vi "PH_VacuumControl.panel.vi"(0 "object ref":refnum<vi>, 5 "error in (no error)":errorcluster) -> (19 "error out":errorcluster)   [LabVIEW 2014, in "PH_VacuumControl.lvlib"]
doc: "By this VI a ross relais can be monitored and switched. \n\nThe indicators \"CLOSED\", \"OPEN\" and \"SWITCH STATE\" show the value of the Beckhoff-Tag: blue indicates bad tag status reference problems, darkgreen false and lightgreen on. If everything is working fine, \"CLOSED\" and \"SWITCH STATE\" should show the same value, while \"OPEN\" has the opposite value. \n\nThe oval button switches the ross relais. It should be in the same state as the \"SWITCH STATE\" indicator. \n\n\"EXIT\" closes the front panel (GUI), while \"Delete Instance\" disconnects and removes the instance from the PCS.\n\nThis VI has no machine safety relevant logig: there is neither a check of internal conclict nor with other objects, for example conflict with other ross relais. Therefore it must be handled with care and should be operated by well educated operators only. It is forseen exclusively for direct operating and testing of the system. \n\nLicense Agreement for this software:\n\nCopyright (C)\nGesellschaft für Schwerionenforschung, GSI\nPlanckstr. 1\n64291 Darmstadt\nGermany\n\nContact: D.Beck@gsi.de \n\nThis program is free software; you can redistribute it and/or modify it under the terms of the GNU General Public License as published by the Free Software Foundation; either version 2 of the license, or (at your option) any later version.\n\nThis program is distributed in the hope that it will be useful, but WITHOUT ANYW ARRANTY; without even the implied warranty of MERCHANTABILITY or FITNESS FOR A PARTICULAR PURPOSE. See the GNU General License for more details (http://www.gnu.org).\n\nGesellschaft für Schwerionenforschung, GSI\nPlanckstr. 1, 64291 Darmstadt, Germany\nFor all questions and ideas contact: M.Richter@gsi.de, H.Brand@gsi.de or D.Beck@gsi.de.\nLast update: 18-DEC-2002"
uses:
  PH_VacuumControl.lvlib
  PH_VacuumControl.Channels.ctl
  CS_Core/CSObj/CSObj.lvlib
  CS_Core/CSSystem/CSSystemLib/CSSystemLib.lvlib
  PH_Basics/PH_Common/PH_Common.lvlib
  PH_Basics/PH_Class/PH_Class.lvlib
  PH_Basics/PH_PSDBWriter/PH_PSDBWriter.lvlib
panel:
  in  "Tab Control":enum32{"Main", "Trending", "Multitrending"}(tab)
  out "Channels":T1={"Channel 1"=99999.0, "Channel 2"=99999.0, "Channel 3"=99999.0, "Channel 4"=99999.0, "Channel 5"=99999.0, "Channel 6"=99999.0, "Name Channel 1"="", "Name Channel 2"="", "Name Channel 3"="", "Name Channel 4"="", "Name Channel 5"="", "Name Channel 6"="", "Upper Limit"=0.0, "Upper Limit 2"=0.0, "Upper Limit 3"=0.0, "Upper Limit 4"=0.0, "Upper Limit 5"=0.0, "Upper Limit 6"=0.0} {"Upper Limit 6" format="%.4e"; "Upper Limit 5" format="%.4e"; "Upper Limit 4" format="%.4e"; "Upper Limit 3" format="%.4e"; "Upper Limit 2" format="%.4e"; "Upper Limit" format="%.4e"; "Channel 6" format="%.4e"; "Channel 5" format="%.4e"; "Channel 4" format="%.4e"; "Channel 3" format="%.4e"; "Channel 2" format="%.4e"; "Channel 1" format="%.4e"}
  in  "Logarithmic":bool
  in  "Channel Name":u16(ring) items=["1"=0, "2"=1, "3"=2, "6"=5, "7"=6]
  out "Trend":cluster{i32[], "Data":dbl[]}[](graph)
  out "Limit reached @":timestamp
  in  "Channel Name 2 MT":u16(ring) caption="Channel Name 2" items=["1"=0, "2"=1, "3"=2, "6"=5, "7"=6]
  in  "Logarithmic MT":bool caption="Logarithmic"
  in  "Channel Name 1 MT":u16(ring) caption="Channel Name 1" items=["1"=0, "2"=1, "3"=2, "6"=5, "7"=6]
  out "Trend MT":cluster{i32[], "Data":dbl[]}[](graph)
  out "Limit reached MT":timestamp caption="Limit reached"
  out "PSDB Status":u32(colorbox)=6618880 caption="PSDB"
  out "State":u32(colorbox) caption="Status"
  out "Device found":bool
  out "Busy":bool
  in  "Set Unit":i32(ring)=1 items=["mBar", "Pascal", "Torr"]
  in  "Delete":bool
  in  "Exit":bool
  # "PCS"
  # "3.40"
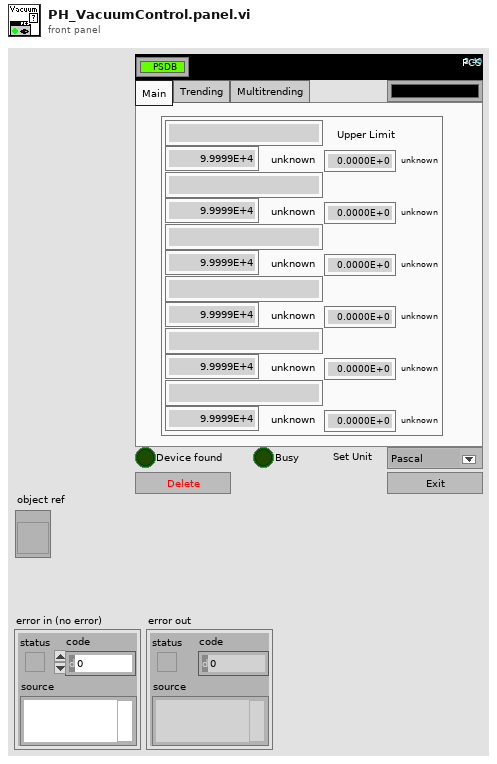
[diagram p1: front panel]
types:
  T1 = typedef "PH_VacuumControl.lvlib/PH_VacuumControl.Channels.ctl" = cluster{"Channel 1":dbl, "Channel 2":dbl, "Channel 3":dbl, "Channel 4":dbl, "Channel 5":dbl, "Channel 6":dbl, "Name Channel 1":string, "Name Channel 2":string, "Name Channel 3":string, "Name Channel 4":string, "Name Channel 5":string, "Name Channel 6":string, "Upper Limit":dbl, "Upper Limit 2":dbl, "Upper Limit 3":dbl, "Upper Limit 4":dbl, "Upper Limit 5":dbl, "Upper Limit 6":dbl}
  T2 = typedef "LVCursorListTypeDef.ctl" = cluster{"Name":string, "Color":u32, "Style":u8, "Point Style":u8, "Name Visible":bool, "Allow Drag":bool, "Cursor Mode":u32, "Plot":i32, "Index":i32, "Position":cluster{"X":dbl, "Y":dbl}, "X Scale":u32, "Y Scale":u32, "Watch Plots":i32[], "Watch All Plots":bool, "Plot Area":i32, "Label Offset":cluster{"X":dbl, "Y":dbl}}[]
  T3 = typedef "PH_VacuumControl.lvlib/PH_VacuumControl.i attribute.ctl" = cluster{"GUI Refs":cluster{"Exit":refnum<vi>, "Set Unit":refnum<vi>, "Device found":refnum<vi>, "Busy":refnum<vi>, "State":refnum<vi>, "Delete":refnum<vi>, "Channels":refnum<vi>, "Channel Name":refnum<vi>, "Trend":refnum<vi>, "Logarithmic":refnum<vi>, "Limit reached":refnum<vi>, "Channel Name 1 MT":refnum<vi>, "Channel Name 2 MT":refnum<vi>, "Trend MT":refnum<vi>, "Logarithmic MT":refnum<vi>, "Limit reached MT":refnum<vi>}, "Device found":bool, "Busy":bool, "Selected Unit":i32, "Channels [mbar]":T1, "Channel Names":cluster{"Channel 1":string, "Channel 2":string, "Channel 3":string, "Channel 4":string, "Channel 5":string, "Channel 6":string}, "Status":T4, "AGCxxx VISA Cluster":T5, "Instr Firmware Revision":string, "Service IDs Pressure":cluster{"Channel 1":i32, "Channel 2":i32, "Channel 3":i32, "Channel 4":i32, "Channel 5":i32, "Channel 6":i32}, "Service IDs Limits":cluster{"Channel 1":i32, "Channel 2":i32, "Channel 3":i32, "Channel 4":i32, "Channel 5":i32, "Channel 6":i32}, "Trend":cluster{"Start Point":timestamp, "Pressures [mbar] Channel 1":dbl[], "Pressures [mbar] Channel 2":dbl[], "Pressures [mbar] Channel 3":dbl[], "Pressures [mbar] Channel 4":dbl[], "Pressures [mbar] Channel 5":dbl[], "Pressures [mbar] Channel 6":dbl[], "Timebase [s]":i32[], "Trend Channel":u16, "Start Fit":dbl, "Trend Channel 1 MT":u16, "Trend Channel 2 MT":u16, "Start or continue Fit MT":dbl, "Continue or start Fit MT":dbl, "Datasets strored":i32, "Dataarray Size":i32}, "Running":bool}
  T4 = typedef "PH_StatusHandler.lvlib/PH_StatusHandler.Status.ctl" = i16
  T5 = typedef "AGCxxx - Driver.lvlib/AGCxxx VISA Control.ctl" = cluster{"VISA resource name":refnum<visa-resource-name>, "VISA Timeout Value (1000 ms)":u32, "Lock Timeout (1000 ms)":u32, "MAX Channel (6)":i32}
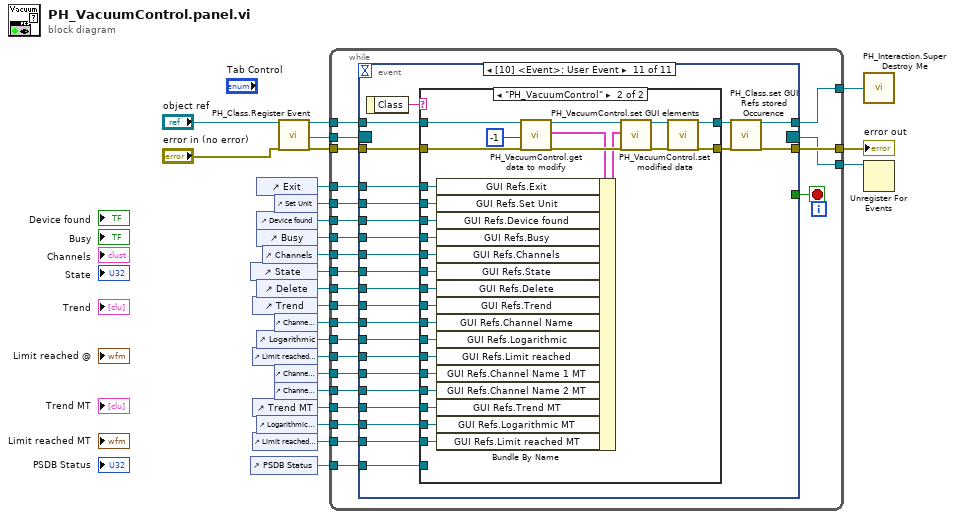
[diagram p0: block diagram]
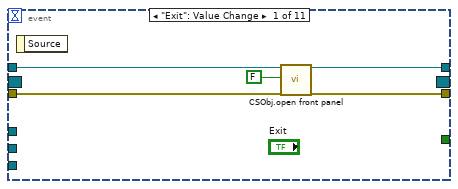
[diagram p2: hidden frame]
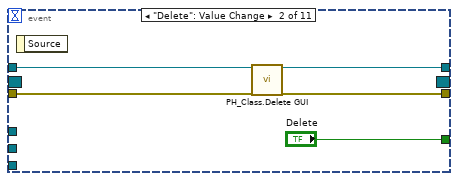
[diagram p3: hidden frame]
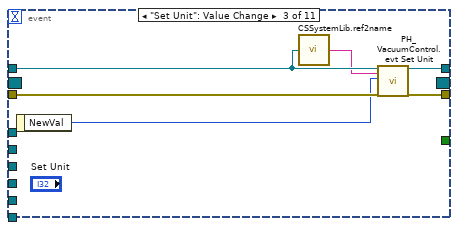
[diagram p4: hidden frame]
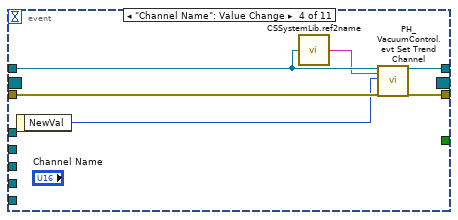
[diagram p5: hidden frame]
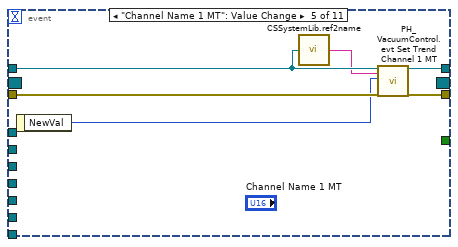
[diagram p6: hidden frame]
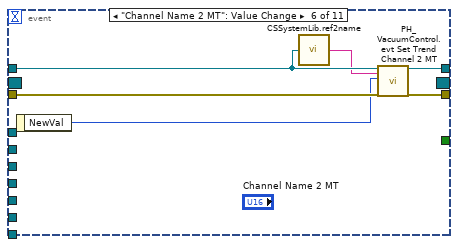
[diagram p7: hidden frame]
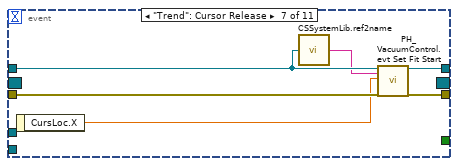
[diagram p8: hidden frame]
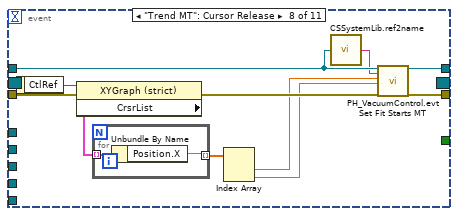
[diagram p9: hidden frame]
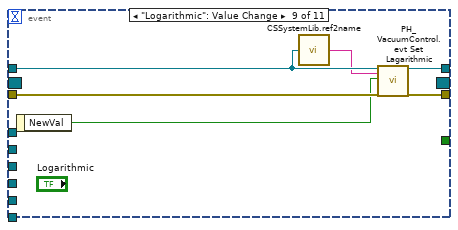
[diagram p10: hidden frame]
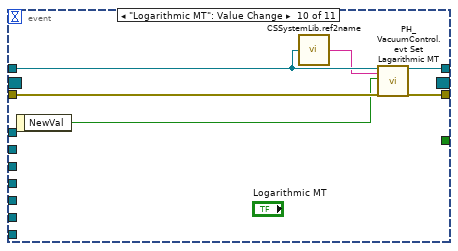
[diagram p11: hidden frame]
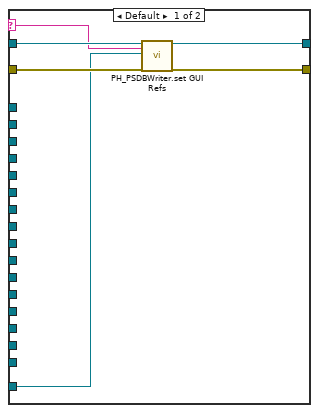
[diagram p12: hidden frame]
diagram:
  n1 = control-ref of="State"() -> (w11:refnum<vi>)
  n2 = control-ref of="PSDB Status"() -> (w17:refnum<vi>)
  n3 = control-ref of="Trend"() -> (w9:refnum<vi>)
  n4 = control-ref of="Limit reached @"() -> (w6:refnum<vi>)
  n5 = control-ref of="Trend MT"() -> (w3:refnum<vi>)
  n6 = control-ref of="Limit reached MT"() -> (w1:refnum<vi>)
  n7 = control-ref of="Exit"() -> (w16:refnum<vi>)
  n8 = control-ref of="Device found"() -> (w14:refnum<vi>)
  n9 = control-ref of="Busy"() -> (w13:refnum<vi>)
  n10 = control-ref of="Delete"() -> (w10:refnum<vi>)
  n11 = control-ref of="Logarithmic"() -> (w7:refnum<vi>)
  n12 = control-ref of="Logarithmic MT"() -> (w2:refnum<vi>)
  n13 = control-ref of="Channels"() -> (w12:refnum<vi>)
  n14 = control-ref of="Set Unit"() -> (w15:refnum<vi>)
  n15 = control-ref of="Channel Name"() -> (w8:refnum<vi>)
  n16 = control-ref of="Channel Name 1 MT"() -> (w5:refnum<vi>)
  n17 = control-ref of="Channel Name 2 MT"() -> (w4:refnum<vi>)
  n18 = call "PH_Class.Register Event.vi"("i ref in"="object ref", "error in (no error)"="error in (no error)") -> ("i ref out"=w23:refnum<vi>, "Event Registration Refnum"=w21:refnum<event-registration>, "error out"=w22:errorcluster)  [unwired: 15 in]
  n19 = while {
    tunnel: w23 -> [w46]
    tunnel: [w45] -> w25
    tunnel: w22 -> [w48]
    tunnel: [w47] -> w24
    tunnel: w21 -> [w44]
    tunnel: [w43] -> w20
    tunnel: w17 -> [w42]
    tunnel: w16 -> [w41]
    tunnel: w15 -> [w40]
    tunnel: w14 -> [w39]
    tunnel: w13 -> [w38]
    tunnel: w12 -> [w37]
    tunnel: w11 -> [w36]
    tunnel: w10 -> [w35]
    tunnel: w9 -> [w34]
    tunnel: w8 -> [w33]
    tunnel: w7 -> [w32]
    tunnel: w6 -> [w31]
    tunnel: w5 -> [w30]
    tunnel: w4 -> [w29]
    tunnel: w3 -> [w28]
    tunnel: w2 -> [w27]
    tunnel: w1 -> [w26]
    stop <- w49 stop-if-true
    n20 = event shown="[10] <Event>: User Event" {
      selector: w44 -> [_ _ _ _ _ _ _ _ _ _ _]
      dyn-events: [_ _ _ _ _ _ _ _ _ _ _] -> w43
      timeout: _ -> [_ _ _ _ _ _ _ _ _ _ _]
      tunnel: [_ "Delete" _ _ _ _ _ _ _ _ _] -> w49
      tunnel: w46 -> [w54 w58 w65 w71 w77 w83 w89 w100 w108 w114 w136]
      tunnel: w48 -> [w52 w57 w63 w69 w75 w81 w87 w96 w106 w112 w135]
      tunnel: [w51 w56 w62 w68 w74 w80 w86 w98 w105 w111 w137] -> w47
      tunnel: [w50 w55 w64 w70 w76 w82 w88 w99 w107 w113 w138] -> w45
      tunnel: w42 -> [_ _ _ _ _ _ _ _ _ _ w131]
      tunnel: w41 -> [_ _ _ _ _ _ _ _ _ _ w130]
      tunnel: w40 -> [_ _ _ _ _ _ _ _ _ _ w129]
      tunnel: w39 -> [_ _ _ _ _ _ _ _ _ _ w128]
      tunnel: w38 -> [_ _ _ _ _ _ _ _ _ _ w127]
      tunnel: w37 -> [_ _ _ _ _ _ _ _ _ _ w126]
      tunnel: w36 -> [_ _ _ _ _ _ _ _ _ _ w125]
      tunnel: w35 -> [_ _ _ _ _ _ _ _ _ _ w124]
      tunnel: w34 -> [_ _ _ _ _ _ _ _ _ _ w123]
      tunnel: w33 -> [_ _ _ _ _ _ _ _ _ _ w122]
      tunnel: w32 -> [_ _ _ _ _ _ _ _ _ _ w121]
      tunnel: w31 -> [_ _ _ _ _ _ _ _ _ _ w120]
      tunnel: w30 -> [_ _ _ _ _ _ _ _ _ _ w119]
      tunnel: w29 -> [_ _ _ _ _ _ _ _ _ _ w118]
      tunnel: w28 -> [_ _ _ _ _ _ _ _ _ _ w117]
      tunnel: w27 -> [_ _ _ _ _ _ _ _ _ _ w116]
      tunnel: w26 -> [_ _ _ _ _ _ _ _ _ _ w115]
      event "Exit": Value Change {
        n21 = event-data() -> ()  [unwired: 1 in, 1 out]
        n22 = call "CSObj.open front panel.vi"("i ref in"=w54, "frontPanelOpen"=FALSE ("front panel open"), "error in (no error)"=w52) -> ("i ref out"=w50:refnum<vi>, "error out"=w51:errorcluster)  [unwired: 15 in]
      }
      event "Delete": Value Change {
        n23 = event-data() -> ()  [unwired: 1 in, 1 out]
        n24 = call "PH_Class.Delete GUI.vi"("VI in"=w58, "error in (no error)"=w57) -> ("VI out"=w55:refnum<vi>, "error out"=w56:errorcluster)  [unwired: 16 in]
      }
      event "Set Unit": Value Change {
        n25 = event-data() -> ("NewVal"=w60:i32)  [unwired: 1 in]
        n26 = call "CSSystemLib.ref2name.vi"("obj refnum"=w65) -> ("name"=w61:string)
        n27 = call "PH_VacuumControl.evt Set Unit.vi"("i ref in"=w65, "Instance"=w61, "Unit"=w60, "error in (no error)"=w63) -> ("i ref out"=w64:refnum<vi>, "error out"=w62:errorcluster)  [unwired: 14 in]
      }
      event "Channel Name": Value Change {
        n28 = event-data() -> ("NewVal"=w66:u16)  [unwired: 1 in]
        n29 = call "CSSystemLib.ref2name.vi"("obj refnum"=w71) -> ("name"=w67:string)
        n30 = call "PH_VacuumControl.evt Set Trend Channel.vi"("i ref in"=w71, "Instance"=w67, "Channel Name"=w66, "error in (no error)"=w69) -> ("i ref out"=w70:refnum<vi>, "error out"=w68:errorcluster)  [unwired: 14 in]
      }
      event "Channel Name 1 MT": Value Change {
        n31 = event-data() -> ("NewVal"=w72:u16)  [unwired: 1 in]
        n32 = call "CSSystemLib.ref2name.vi"("obj refnum"=w77) -> ("name"=w73:string)
        n33 = call "PH_VacuumControl.evt Set Trend Channel 1 MT.vi"("i ref in"=w77, "Instance"=w73, "Channel Name 1 MT"=w72, "error in (no error)"=w75) -> ("i ref out"=w76:refnum<vi>, "error out"=w74:errorcluster)  [unwired: 14 in]
      }
      event "Channel Name 2 MT": Value Change {
        n34 = event-data() -> ("NewVal"=w78:u16)  [unwired: 1 in]
        n35 = call "CSSystemLib.ref2name.vi"("obj refnum"=w83) -> ("name"=w79:string)
        n36 = call "PH_VacuumControl.evt Set Trend Channel 2 MT.vi"("i ref in"=w83, "Instance"=w79, "Channel Name 2 MT"=w78, "error in (no error)"=w81) -> ("i ref out"=w82:refnum<vi>, "error out"=w80:errorcluster)  [unwired: 14 in]
      }
      event "Trend": Cursor Release {
        n37 = event-data() -> ("CursLoc.X"=w84:dbl)  [unwired: 1 in]
        n38 = call "CSSystemLib.ref2name.vi"("obj refnum"=w89) -> ("name"=w85:string)
        n39 = call "PH_VacuumControl.evt Set Fit Start.vi"("i ref in"=w89, "Instance"=w85, "Fit Start"=w84, "error in (no error)"=w87) -> ("i ref out"=w88:refnum<vi>, "error out"=w86:errorcluster)  [unwired: 14 in]
      }
      event "Trend MT": Cursor Release {
        n40 = event-data() -> ("CtlRef"=w94:refnum<vi>)  [unwired: 1 in]
        n41 = property class="XYGraph (strict)"(reference=w94, error in=w96) -> (error out=w95:errorcluster, "CrsrList"=w93:T2)  [unwired: 1 out]
        n42 = for {
          tunnel: w93 -> [w102] mode=indexing
          tunnel: [w101] -> w92 mode=indexing
          n43 = Unbundle By Name(w102) -> ("Position.X"=w101:dbl)
        }
        n44 = Index Array(array=w92) -> (element #1=w91:dbl, element #2=w90:dbl)  [unwired: 2 in]
        n45 = call "CSSystemLib.ref2name.vi"("obj refnum"=w100) -> ("name"=w97:string)
        n46 = call "PH_VacuumControl.evt Set Fit Starts MT.vi"("i ref in"=w100, "Instance"=w97, "Start Fit MT"=w91, "Continue Fit MT"=w90, "error in (no error)"=w95) -> ("i ref out"=w99:refnum<vi>, "error out"=w98:errorcluster)  [unwired: 13 in]
      }
      event "Logarithmic": Value Change {
        n47 = event-data() -> ("NewVal"=w103:bool)  [unwired: 1 in]
        n48 = call "CSSystemLib.ref2name.vi"("obj refnum"=w108) -> ("name"=w104:string)
        n49 = call "PH_VacuumControl.evt Set Lagarithmic.vi"("i ref in"=w108, "Instance"=w104, "Logarithmic?"=w103, "error in (no error)"=w106) -> ("i ref out"=w107:refnum<vi>, "error out"=w105:errorcluster)  [unwired: 14 in]
      }
      event "Logarithmic MT": Value Change {
        n50 = event-data() -> ("NewVal"=w109:bool)  [unwired: 1 in]
        n51 = call "CSSystemLib.ref2name.vi"("obj refnum"=w114) -> ("name"=w110:string)
        n52 = call "PH_VacuumControl.evt Set Lagarithmic MT.vi"("i ref in"=w114, "Instance"=w110, "MT Logarithmic?"=w109, "error in (no error)"=w112) -> ("i ref out"=w113:refnum<vi>, "error out"=w111:errorcluster)  [unwired: 14 in]
      }
      event User Event {
        n53 = event-data() -> ("Class"=w132:string)  [unwired: 1 in]
        n54 = case shown="\"PH_VacuumControl\"" w132 {
          selector: w132 -> [w140 _]
          tunnel: w136 -> [w144 w166]
          tunnel: w135 -> [w142 w165]
          tunnel: [w143 w145] -> w134
          tunnel: [w141 w146] -> w133
          tunnel: w131 -> [w139 _]
          tunnel: w130 -> [_ w164]
          tunnel: w129 -> [_ w163]
          tunnel: w128 -> [_ w162]
          tunnel: w127 -> [_ w161]
          tunnel: w126 -> [_ w160]
          tunnel: w125 -> [_ w159]
          tunnel: w124 -> [_ w158]
          tunnel: w123 -> [_ w157]
          tunnel: w122 -> [_ w156]
          tunnel: w121 -> [_ w155]
          tunnel: w120 -> [_ w154]
          tunnel: w119 -> [_ w153]
          tunnel: w118 -> [_ w152]
          tunnel: w117 -> [_ w151]
          tunnel: w116 -> [_ w150]
          tunnel: w115 -> [_ w149]
          frame Default {
            n55 = call "PH_PSDBWriter.set GUI Refs.vi"("i ref in"=w144, "Class"=w140, "Ref PSDB Status"=w139, "error in"=w142) -> ("i ref out"=w143:refnum<vi>, "error out"=w141:errorcluster)  [unwired: 14 in]
          }
          frame "PH_VacuumControl" {
            n56 = call "PH_VacuumControl.get data to modify.vi"("i ref in"=w166, "ms timeout (10000)"=-1, "error in (no error)"=w165) -> ("i ref out"=w171:refnum<vi>, "i attribute"=w168:T3, "error out"=w170:errorcluster)  [unwired: 13 in, 1 out]
            n57 = Bundle By Name(cluster=w168, "GUI Refs.Exit"=w164, "GUI Refs.Set Unit"=w163, "GUI Refs.Device found"=w162, "GUI Refs.Busy"=w161, "GUI Refs.Channels"=w160, "GUI Refs.State"=w159, "GUI Refs.Delete"=w158, "GUI Refs.Trend"=w157, "GUI Refs.Channel Name"=w156, "GUI Refs.Logarithmic"=w155, "GUI Refs.Limit reached"=w154, "GUI Refs.Channel Name 1 MT"=w153, "GUI Refs.Channel Name 2 MT"=w152, "GUI Refs.Trend MT"=w151, "GUI Refs.Logarithmic MT"=w150, "GUI Refs.Limit reached MT"=w149) -> (w167:T3)
            n58 = call "PH_VacuumControl.set modified data.vi"("i ref in"=w171, "i attribute"=w167, "error in (no error)"=w170) -> ("i ref out"=w147:refnum<vi>, "error out"=w148:errorcluster)  [unwired: 15 in]
            n59 = call "PH_VacuumControl.set GUI elements.vi"("i ref in"=w147, "error in (no error)"=w148) -> ("i ref out"=w145:refnum<vi>, "error out"=w146:errorcluster)  [unwired: 16 in]
          }
        }
        n60 = call "PH_Class.set GUI Refs stored Occurence.vi"("i ref in"=w134, "error in (no error)"=w133) -> ("i ref out"=w138:refnum<vi>, "error out"=w137:errorcluster)  [unwired: 16 in]
      }
    }
  }
  "error out" <- w24
  n61 = call "PH_Interaction.Super Destroy Me.vi"("i ref out"=w25) -> ()
  n62 = Unregister For Events(event registration refnum=w20) -> ()  [unwired: 1 in, 1 out]
